vi "Data EEPROM Test_v2.vi"(8 "error in (no error)":errorcluster, 11 "ControlBoard VISA":refnum<visa-resource-name>="ControlBoard") -> (0 "error out":errorcluster, 2 "Passed?":string, 3 "Test Result":string)   [LabVIEW 2022 SP3]
uses:
  SupportVIs/VISA Flush IO Buffer Mask.ctl
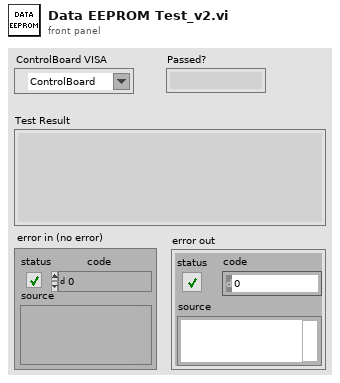
[diagram p1: front panel]
types:
  T1 = typedef "VISA Flush IO Buffer Mask.ctl" = u16
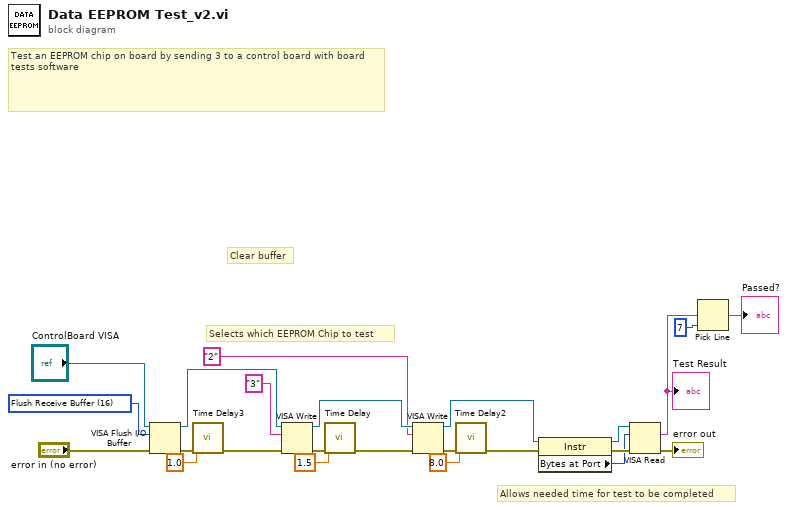
[diagram p0: block diagram]
diagram:
  w23 = T1 16 items=["Flush Receive Buffer"=16, "Write Transmit Buffer to Device"=32, "Flush Receive Buffer (No I/O)"=64, "Flush Transmit Buffer"=128] ("Mask")
  # "Selects which EEPROM Chip to test"
  # "Allows needed time for test to be completed"
  # "Test an EEPROM chip on board by sending 3 to a control board with board tests software"
  # "Clear buffer"
  n1 = VISA Flush I/O Buffer(VISA resource name="ControlBoard VISA", mask (16)=w23, error in (no error)="error in (no error)") -> (VISA resource name out=w21:refnum<visa-resource-name>, error out=w18:errorcluster)
  n2 = call "Time Delay3"("error in (no error)"=w18, "Delay Time (s)"=1.0) -> ("error out"=w17:errorcluster)  [unwired: 9 in]
  n3 = VISA Write(VISA resource name=w21, write buffer="3", error in (no error)=w17) -> (VISA resource name out=w15:refnum<visa-resource-name>, error out=w22:errorcluster)  [unwired: 1 out]
  n4 = call "Time Delay"("error in (no error)"=w22, "Delay Time (s)"=1.5) -> ("error out"=w16:errorcluster)  [unwired: 9 in]
  n5 = VISA Write(VISA resource name=w15, write buffer="2", error in (no error)=w16) -> (VISA resource name out=w12:refnum<visa-resource-name>, error out=w13:errorcluster)  [unwired: 1 out]
  n6 = call "Time Delay2"("error in (no error)"=w13, "Delay Time (s)"=8.0) -> ("error out"=w11:errorcluster)  [unwired: 9 in]
  n7 = property class="Instr"(reference=w12, error in=w11) -> (reference out=w10:refnum<visa-resource-name>, error out=w9:errorcluster, "Bytes at Port"=w8:u32)
  n8 = VISA Read(VISA resource name=w10, byte count=w8, error in (no error)=w9) -> (read buffer=w6:string, error out=→"error out":errorcluster)  [unwired: 2 out]
  "Test Result" <- w6
  n9 = Pick Line(multi-line string=w6, line index=7) -> (output string=→"Passed?":string)  [unwired: 1 in]
